vi "DMSO_load_acid_BM.vi"(6 "COM Port":refnum<visa-resource-name>="COM3", 7 "Pump Parameters":T1={"Speed 1"="100", "Speed 2"="250", "Speed 3"="350", "Speed 4"="250", "UW/Sample"="5", "Sparge"="2", "Std"="4", "Waste"="15", "Air"="14", "Milli-Q"="1", "H2SO4"="6", "NaOH"="3", "Catalyst"="7", "Cell (H+ side)"="8", "Cell (sample side)"="9", "NaCl"="11"}, 9 "step to ml":dbl=1920.0, 10 "Total Vol. (mL)":dbl=10.0, 11 "Sample Vol. (mL)":dbl=10.0) -> ()   [LabVIEW 2021]
panel:
  out "Full Command":string="V100O6P19200O8V250D19200V100O14P3840O8V250D3840V100O1P23040O15V250D23040"
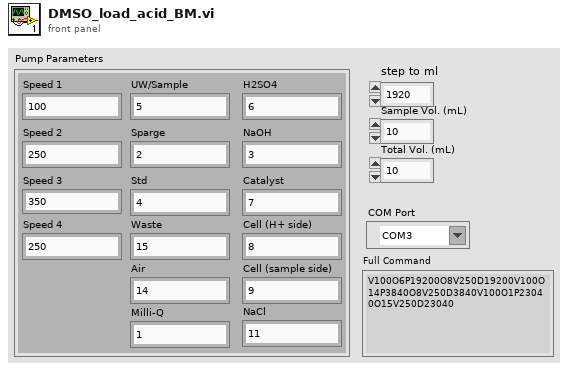
[diagram p1: front panel]
types:
  T1 = cluster{"Speed 1":string, "Speed 2":string, "Speed 3":string, "Speed 4":string, "UW/Sample":string, "Sparge":string, "Std":string, "Waste":string, "Air":string, "Milli-Q":string, "H2SO4":string, "NaOH":string, "Catalyst":string, "Cell (H+ side)":string, "Cell (sample side)":string, "NaCl":string}
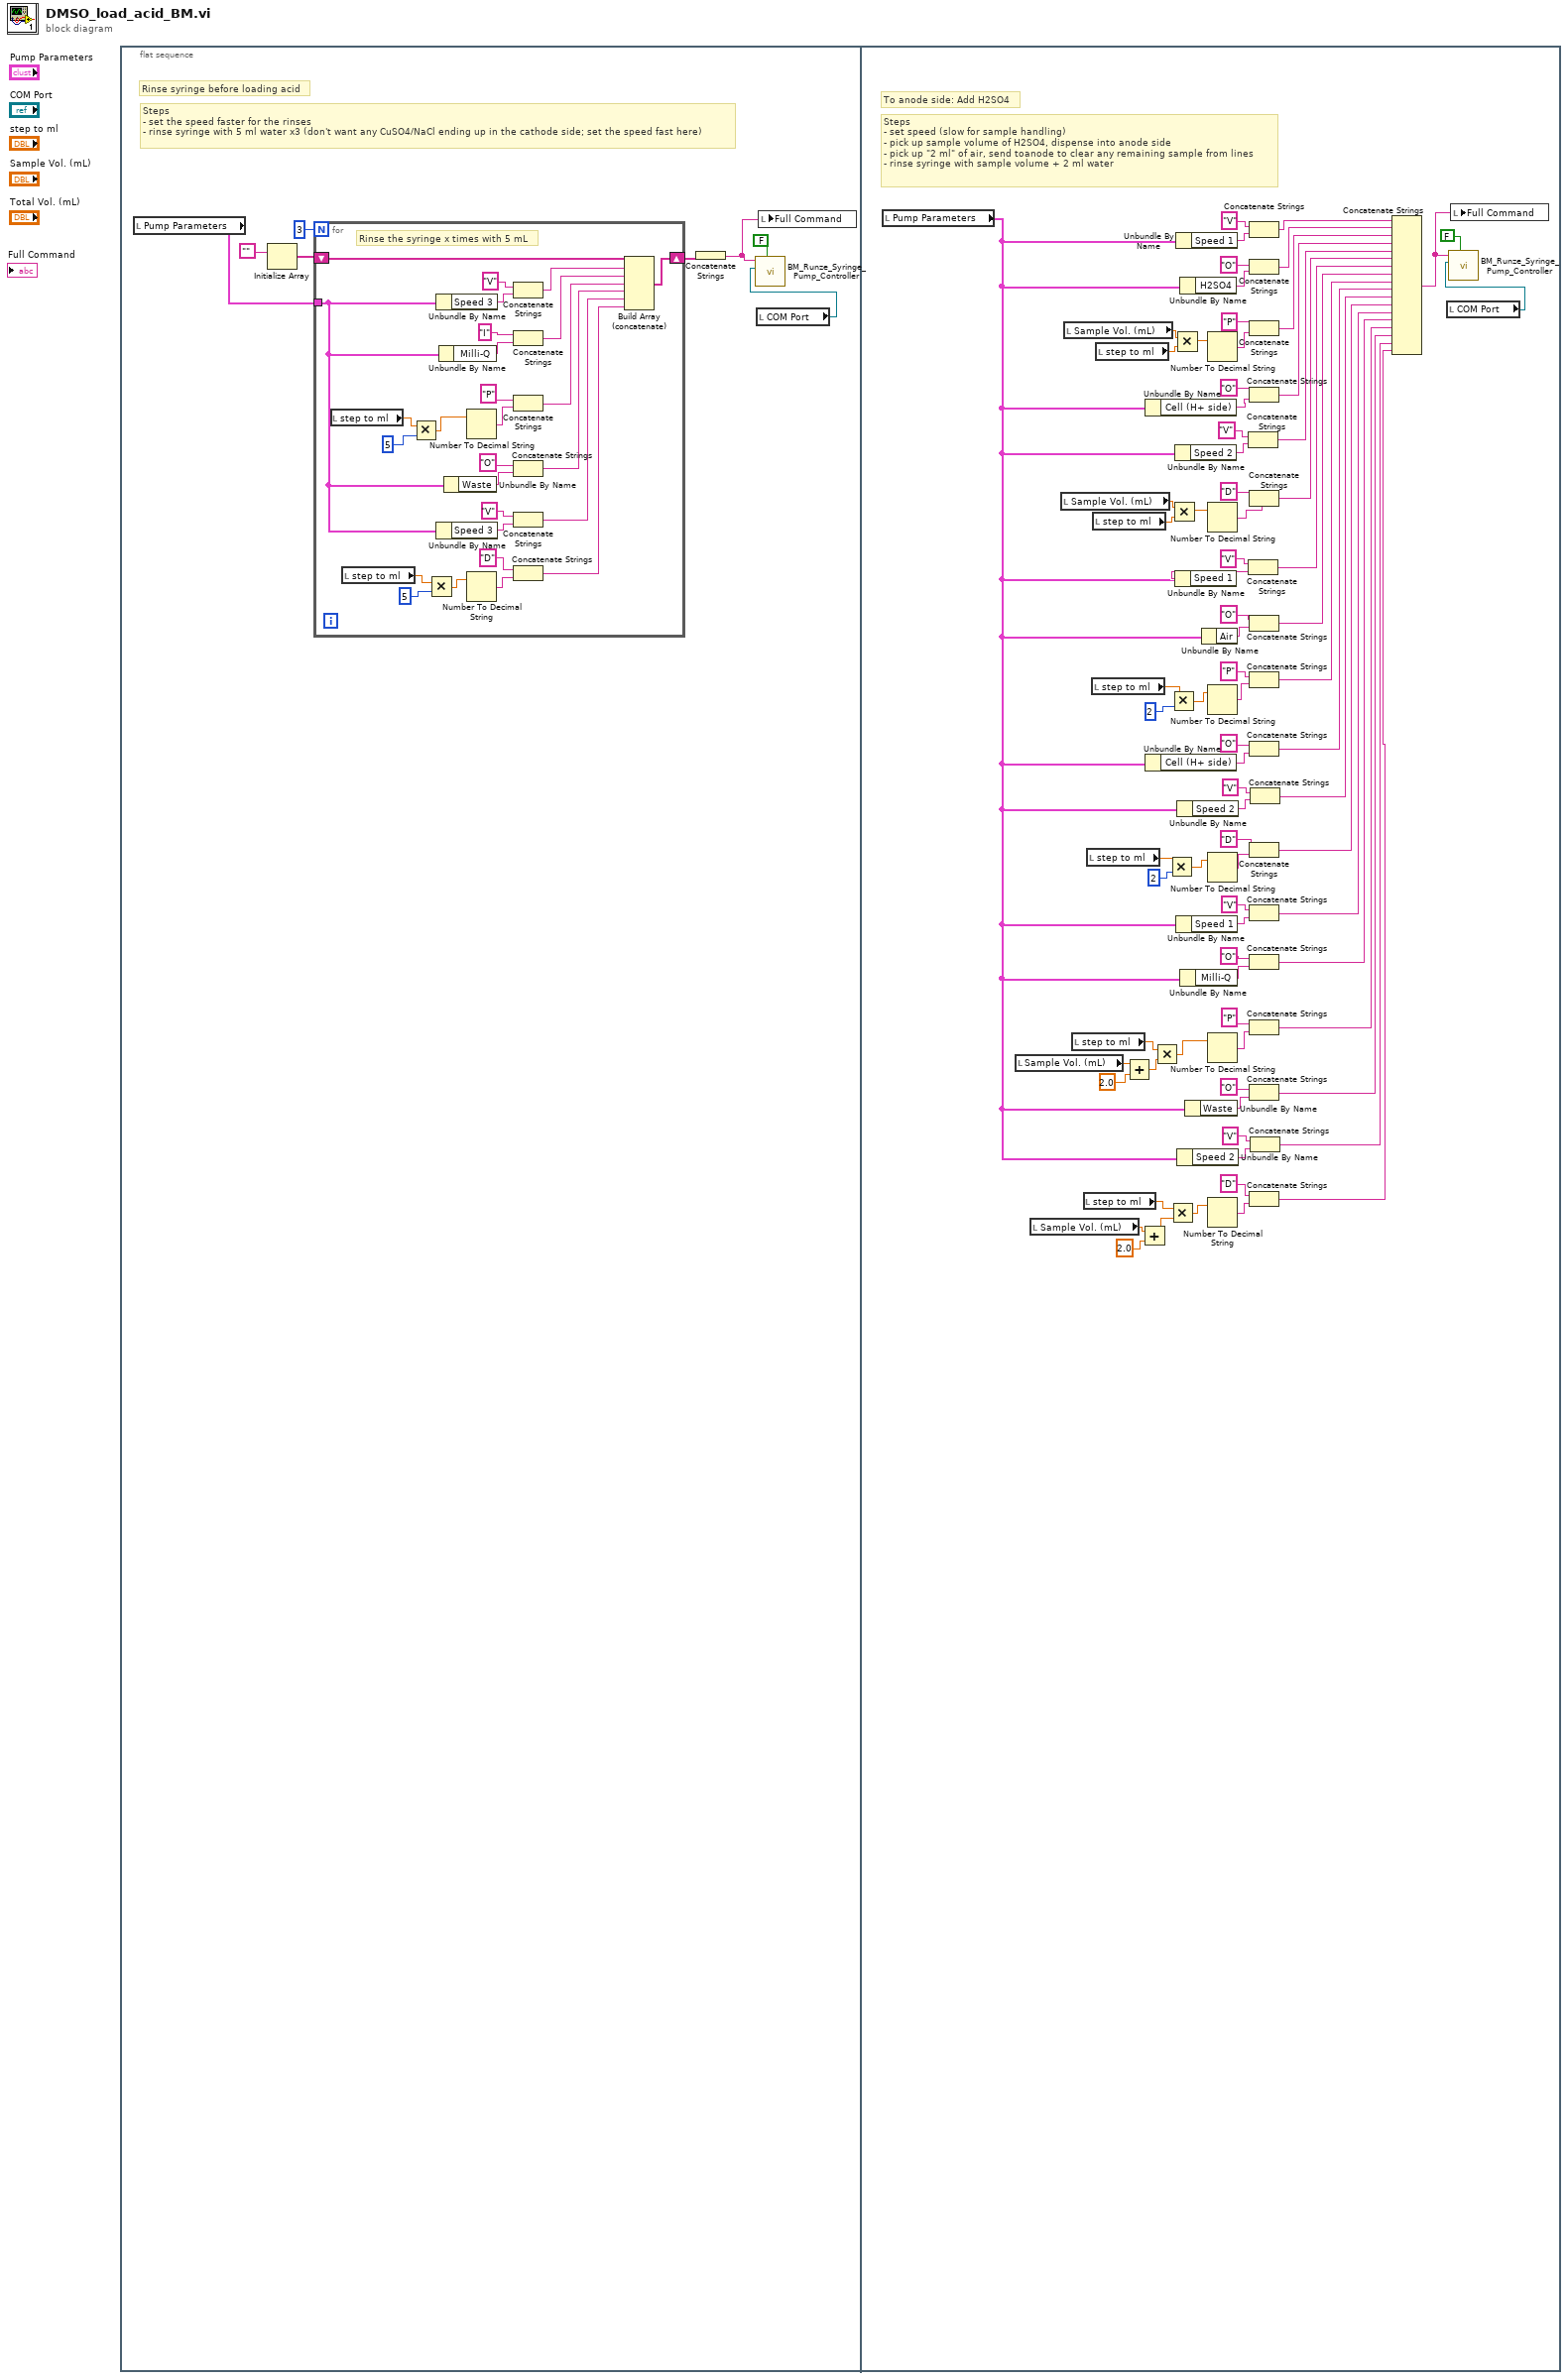
[diagram p0: block diagram]
diagram:
  n1 = flat-sequence {
    frame #0 {
      # "Steps\n- set the speed faster for the rinses\n- rinse syringe with 5 ml water x3 (don't want any CuSO4/NaCl ending up in the cathode side; set the speed fast here)"
      # "Rinse syringe before loading acid"
      n2 = local read "Pump Parameters"() -> (w3:T1)
      n3 = Initialize Array("") -> (w5:string[])  [unwired: 1 in]
      n4 = for {
        N: 3 -> [_]
        shift-right: [w9] -> w4
        shift-left: w5 -> [w35]
        tunnel: w3 -> [w16]
        # "Rinse the syringe x times with 5 mL"
        n5 = local read "step to ml"() -> (w21:dbl)
        n6 = local read "step to ml"() -> (w28:dbl)
        n7 = Multiply(x=w21, y=5) -> (x*y=w17:dbl)
        n8 = Multiply(x=w28, y=5) -> (x*y=w26:dbl)
        n9 = Unbundle By Name(w16) -> ("Speed 3"=w33:string)
        n10 = Unbundle By Name(w16) -> ("Speed 3"=w34:string)
        n11 = Unbundle By Name(w16) -> ("Milli-Q"=w22:string)
        n12 = Unbundle By Name(w16) -> ("Waste"=w23:string)
        n13 = Number To Decimal String(number=w17) -> (decimal integer string=w25:string)  [unwired: 1 out]
        n14 = Number To Decimal String(number=w26) -> (decimal integer string=w29:string)  [unwired: 1 out]
        n15 = Concatenate Strings("V", w33) -> (w15:string)
        n16 = Concatenate Strings("I", w22) -> (w14:string)
        n17 = Concatenate Strings("P", w25) -> (w13:string)
        n18 = Concatenate Strings("O", w23) -> (w12:string)
        n19 = Concatenate Strings("V", w34) -> (w11:string)
        n20 = Concatenate Strings("D", w29) -> (w10:string)
        n21 = Build Array (concatenate)(w35, w15, w14, w13, w12, w11, w10) -> (w9:string[])
      }
      n22 = Concatenate Strings(w4) -> (w1:string)
      n23 = local read "COM Port"() -> (w8:refnum<visa-resource-name>)
      n24 = call "BM_Runze_Syringe_Pump_Controller.vi"("Initialize Plunger?"=FALSE ("Initialize?"), "COM Port (Runze)"=w8, "Enter Command"=w1) -> ()  [unwired: 6 in, 3 out]
      n25 = local write "Full Command"(w1) -> ()
    }
    frame #1 {
      # "Steps\n- set speed (slow for sample handling)\n- pick up sample volume of H2SO4, dispense into anode side\n- pick up \"2 ml\" of air, send toanode to clear any remaining sample from lines\n- rinse syringe with sample volume + 2 ml water"
      # "To anode side: Add H2SO4"
      n26 = local read "Pump Parameters"() -> (w37:T1)
      n27 = local read "Sample Vol. (mL)"() -> (w71:dbl)
      n28 = local read "Sample Vol. (mL)"() -> (w70:dbl)
      n29 = local read "Sample Vol. (mL)"() -> (w73:dbl)
      n30 = local read "Sample Vol. (mL)"() -> (w72:dbl)
      n31 = local read "step to ml"() -> (w87:dbl)
      n32 = local read "step to ml"() -> (w81:dbl)
      n33 = local read "step to ml"() -> (w94:dbl)
      n34 = local read "step to ml"() -> (w98:dbl)
      n35 = local read "step to ml"() -> (w106:dbl)
      n36 = local read "step to ml"() -> (w111:dbl)
      n37 = Add(x=w71, y=2.0) -> (x+y=w67:dbl)
      n38 = Add(x=w70, y=2.0) -> (x+y=w66:dbl)
      n39 = Unbundle By Name(w37) -> ("Cell (H+ side)"=w74:string)
      n40 = Unbundle By Name(w37) -> ("Cell (H+ side)"=w75:string)
      n41 = Multiply(x=w87, y=w67) -> (x*y=w90:dbl)
      n42 = Multiply(x=w94, y=2) -> (x*y=w95:dbl)
      n43 = Multiply(x=w81, y=w66) -> (x*y=w82:dbl)
      n44 = Multiply(x=w98, y=2) -> (x*y=w101:dbl)
      n45 = Multiply(x=w73, y=w106) -> (x*y=w107:dbl)
      n46 = Multiply(x=w72, y=w111) -> (x*y=w112:dbl)
      n47 = Unbundle By Name(w37) -> ("Speed 2"=w65:string)
      n48 = Unbundle By Name(w37) -> ("Speed 1"=w64:string)
      n49 = Unbundle By Name(w37) -> ("Speed 1"=w113:string)
      n50 = Unbundle By Name(w37) -> ("Speed 1"=w59:string)
      n51 = Unbundle By Name(w37) -> ("Speed 2"=w61:string)
      n52 = Unbundle By Name(w37) -> ("Speed 2"=w57:string)
      n53 = Unbundle By Name(w37) -> ("H2SO4"=w78:string)
      n54 = Unbundle By Name(w37) -> ("Milli-Q"=w86:string)
      n55 = Unbundle By Name(w37) -> ("Waste"=w85:string)
      n56 = Unbundle By Name(w37) -> ("Air"=w102:string)
      n57 = Number To Decimal String(number=w112) -> (decimal integer string=w109:string)  [unwired: 1 out]
      n58 = Number To Decimal String(number=w107) -> (decimal integer string=w104:string)  [unwired: 1 out]
      n59 = Number To Decimal String(number=w101) -> (decimal integer string=w96:string)  [unwired: 1 out]
      n60 = Number To Decimal String(number=w95) -> (decimal integer string=w91:string)  [unwired: 1 out]
      n61 = Number To Decimal String(number=w90) -> (decimal integer string=w83:string)  [unwired: 1 out]
      n62 = Number To Decimal String(number=w82) -> (decimal integer string=w80:string)  [unwired: 1 out]
      n63 = Concatenate Strings("V", w65) -> (w51:string)
      n64 = Concatenate Strings("V", w64) -> (w49:string)
      n65 = Concatenate Strings("V", w113) -> (w55:string)
      n66 = Concatenate Strings("O", w78) -> (w54:string)
      n67 = Concatenate Strings("P", w109) -> (w53:string)
      n68 = Concatenate Strings("O", w74) -> (w52:string)
      n69 = Concatenate Strings("D", w104) -> (w50:string)
      n70 = Concatenate Strings("O", w102) -> (w48:string)
      n71 = Concatenate Strings("P", w96) -> (w47:string)
      n72 = Concatenate Strings("O", w75) -> (w46:string)
      n73 = Concatenate Strings("D", w91) -> (w44:string)
      n74 = Concatenate Strings("V", w59) -> (w43:string)
      n75 = Concatenate Strings("O", w86) -> (w42:string)
      n76 = Concatenate Strings("P", w83) -> (w41:string)
      n77 = Concatenate Strings("O", w85) -> (w40:string)
      n78 = Concatenate Strings("D", w80) -> (w38:string)
      n79 = Concatenate Strings("V", w61) -> (w45:string)
      n80 = Concatenate Strings("V", w57) -> (w39:string)
      n81 = Concatenate Strings(w55, w54, w53, w52, w51, w50, w49, w48, w47, w46, w45, w44, w43, w42, w41, w40, w39, w38) -> (w77:string)
      n82 = local read "COM Port"() -> (w76:refnum<visa-resource-name>)
      n83 = call "BM_Runze_Syringe_Pump_Controller.vi"("Initialize Plunger?"=FALSE ("Initialize?"), "COM Port (Runze)"=w76, "Enter Command"=w77) -> ()  [unwired: 6 in, 3 out]
      n84 = local write "Full Command"(w77) -> ()
    }
  }
